vi "Expand.vi"(8 "error in (no error)":errorcluster, 9 "Factor":u64=1, 10 "Input":string, 11 "Galaxy in":refnum<class "Galaxy.lvclass">[](array[class])) -> (0 "error out":errorcluster, 3 "Array":refnum<class "Galaxy.lvclass">[](array[class]))   [LabVIEW 2020, in "Galaxy.lvclass"]
uses:
  Galaxy/Galaxy.lvclass
  Galaxy/Galaxy.lvclass/Galaxy.ctl
  93158617-729e-4cb0-8a79-370734b35a69.vi
  4fc83f36-bdbd-423c-9f43-ae725be9c568.vi
  <vilib>/Comparison/Equal/Equal Functor/Equal Functor.lvclass
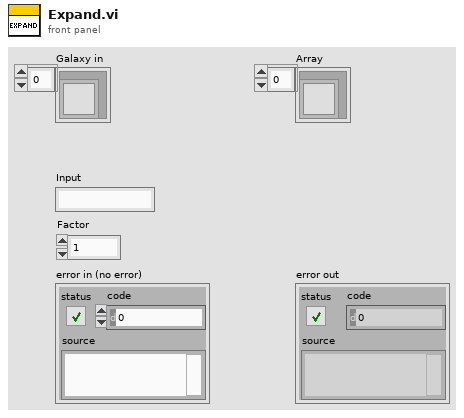
[diagram p1: front panel]
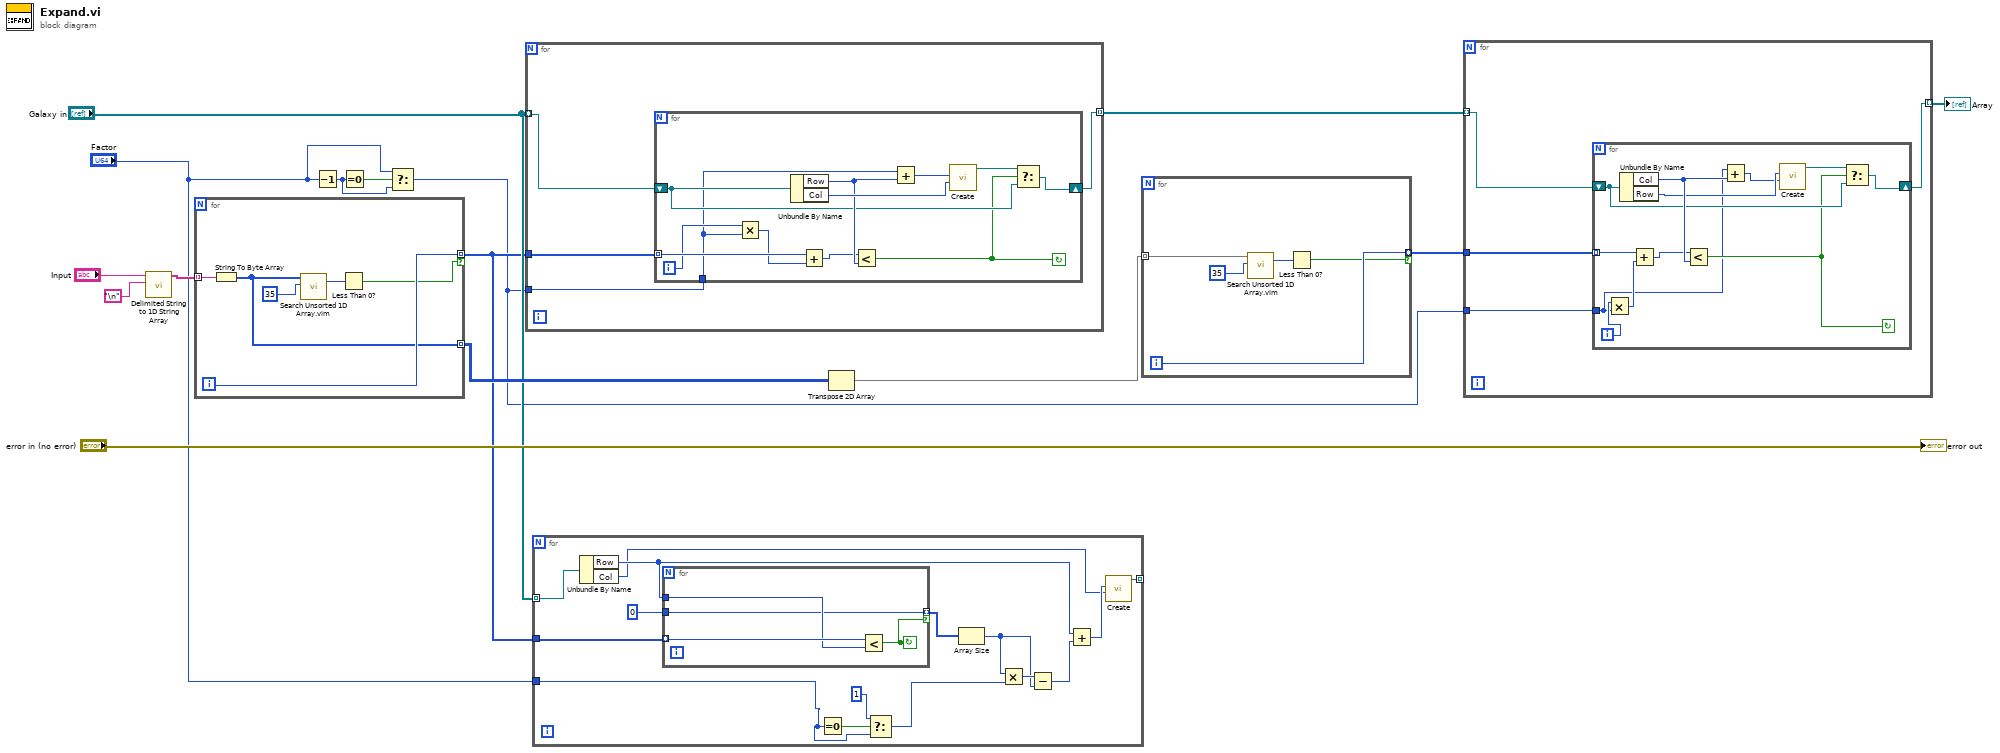
[diagram p0: block diagram]
diagram:
  n1 = call <vilib>:"Delimited String to 1D String Array.vi"("delimiter"="\n", "delimited string"="Input") -> ("string array"=w13:string[])  [unwired: 9 in]
  n2 = for {
    tunnel: w13 -> [w21] mode=indexing
    tunnel: [w18] -> w4 mode=indexing if=w17
    tunnel: [w16] -> w11 mode=indexing
    i -> [w18]
    n3 = String To Byte Array(string=w21) -> (unsigned byte array=w16:u8[])
    n4 = call "Search Unsorted 1D Array.vim"("element"=u8 35 ("y"), "unsorted 1D array"=w16) -> ("index of element"=w19:i32)  [unwired: 9 in]
    n5 = Less Than 0?(x=w19) -> (x < 0?=w17:bool)
  }
  n6 = Decrement(x="Factor") -> (x-1=w6:u64)
  n7 = Equal To 0?(x=w6) -> (x = 0?=w7:bool)
  n8 = Select(t="Factor", s=w7, f=w6) -> (s? t:f=w3:u64)
  n9 = for {
    tunnel: "Galaxy in" -> [w24] mode=indexing
    tunnel: w4 -> [w25]
    tunnel: [w23] -> w2 mode=indexing
    tunnel: w3 -> [w22]
    n10 = for {
      tunnel: w25 -> [w37] mode=indexing
      shift-right: [w31] -> w23
      shift-left: w24 -> [w32]
      tunnel: w22 -> [w26]
      i -> [w28]
      stop <- w30 continue-if-true
      n11 = Multiply(x=w28, y=w26) -> (x*y=w27:u64)
      n12 = Unbundle By Name(w32) -> ("Row"=w34:u64, "Col"=w36:u64)
      n13 = Add(x=w37, y=w27) -> (x+y=w29:u64)
      n14 = Less?(x=w29, y=w34) -> (x < y?=w30:bool)
      n15 = Add(x=w26, y=w34) -> (x+y=w35:u64)
      n16 = call "Create.vi"("Col"=w36, "Row"=w35) -> ("Galaxy"=w33:refnum<class "Galaxy.lvclass">)  [unwired: 8 in, 1 out]
      n17 = Select(t=w33, s=w30, f=w32) -> (s? t:f=w31:refnum<class "Galaxy.lvclass">)
    }
  }
  n18 = for {
    tunnel: "Galaxy in" -> [w51] mode=indexing
    tunnel: w4 -> [w52]
    tunnel: "Factor" -> [w38]
    tunnel: [w46] -> _ mode=indexing
    n19 = Unbundle By Name(w51) -> ("Row"=w50:u64, "Col"=w47:u64)
    n20 = for {
      tunnel: w52 -> [w56] mode=indexing
      tunnel: w50 -> [w55]
      tunnel: [w54] -> w44 mode=indexing if=w53
      tunnel: u64 0 ("Factor") -> [w54]
      stop <- w53 continue-if-true
      n21 = Less?(x=w56, y=w55) -> (x < y?=w53:bool)
    }
    n22 = Equal To 0?(x=w38) -> (x = 0?=w41:bool)
    n23 = Select(t=u64 1, s=w41, f=w38) -> (s? t:f=w39:u64)
    n24 = Array Size(array=w44) -> (size(s)=w42:i32)
    n25 = Multiply(x=w42, y=w39) -> (x*y=w49:u64)
    n26 = Subtract(x=w49, y=w42) -> (x-y=w43:u64)
    n27 = Add(x=w50, y=w43) -> (x+y=w48:u64)
    n28 = call "Create.vi"("Col"=w47, "Row"=w48) -> ("Galaxy"=w46:refnum<class "Galaxy.lvclass">)  [unwired: 8 in, 1 out]
  }
  n29 = Transpose 2D Array(2D array=w11) -> (transposed array=w10:u8[][])
  n30 = for {
    tunnel: w10 -> [w57] mode=indexing
    tunnel: [w59] -> w8 mode=indexing if=w58
    i -> [w59]
    n31 = call "Search Unsorted 1D Array.vim"("element"=u8 35 ("y"), "unsorted 1D array"=w57) -> ("index of element"=w60:i32)  [unwired: 9 in]
    n32 = Less Than 0?(x=w60) -> (x < 0?=w58:bool)
  }
  n33 = for {
    tunnel: w2 -> [w64] mode=indexing
    tunnel: w8 -> [w65]
    tunnel: [w63] -> w9 mode=indexing
    tunnel: w3 -> [w62]
    n34 = for {
      tunnel: w65 -> [w77] mode=indexing
      shift-right: [w73] -> w63
      shift-left: w64 -> [w74]
      tunnel: w62 -> [w66]
      i -> [w68]
      stop <- w72 continue-if-true
      n35 = Multiply(x=w68, y=w66) -> (x*y=w67:u64)
      n36 = Unbundle By Name(w74) -> ("Col"=w76:u64, "Row"=w71:u64)
      n37 = Add(x=w77, y=w67) -> (x+y=w69:u64)
      n38 = Less?(x=w69, y=w76) -> (x < y?=w72:bool)
      n39 = Add(x=w66, y=w76) -> (x+y=w70:u64)
      n40 = call "Create.vi"("Col"=w70, "Row"=w71) -> ("Galaxy"=w75:refnum<class "Galaxy.lvclass">)  [unwired: 8 in, 1 out]
      n41 = Select(t=w75, s=w72, f=w74) -> (s? t:f=w73:refnum<class "Galaxy.lvclass">)
    }
  }
  "Array" <- w9
  "error out" <- "error in (no error)"
